vi "Open file in table.vi"() -> (0 "Error Out":errorcluster, 1 "Command Array":dbl[][](array[numeric]), 2 "Command Table":string[][](table), 3 "Details":string, 5 "Original Array":dbl[][](array[numeric]))   [LabVIEW 2011]
uses:
  <vilib>/Utility/file.llb/Read From Spreadsheet File (string).vi
panel:
  out "cancelled":bool
  out "Original Table":string[][](table)
  out "reversed array":i32[](array[numeric])
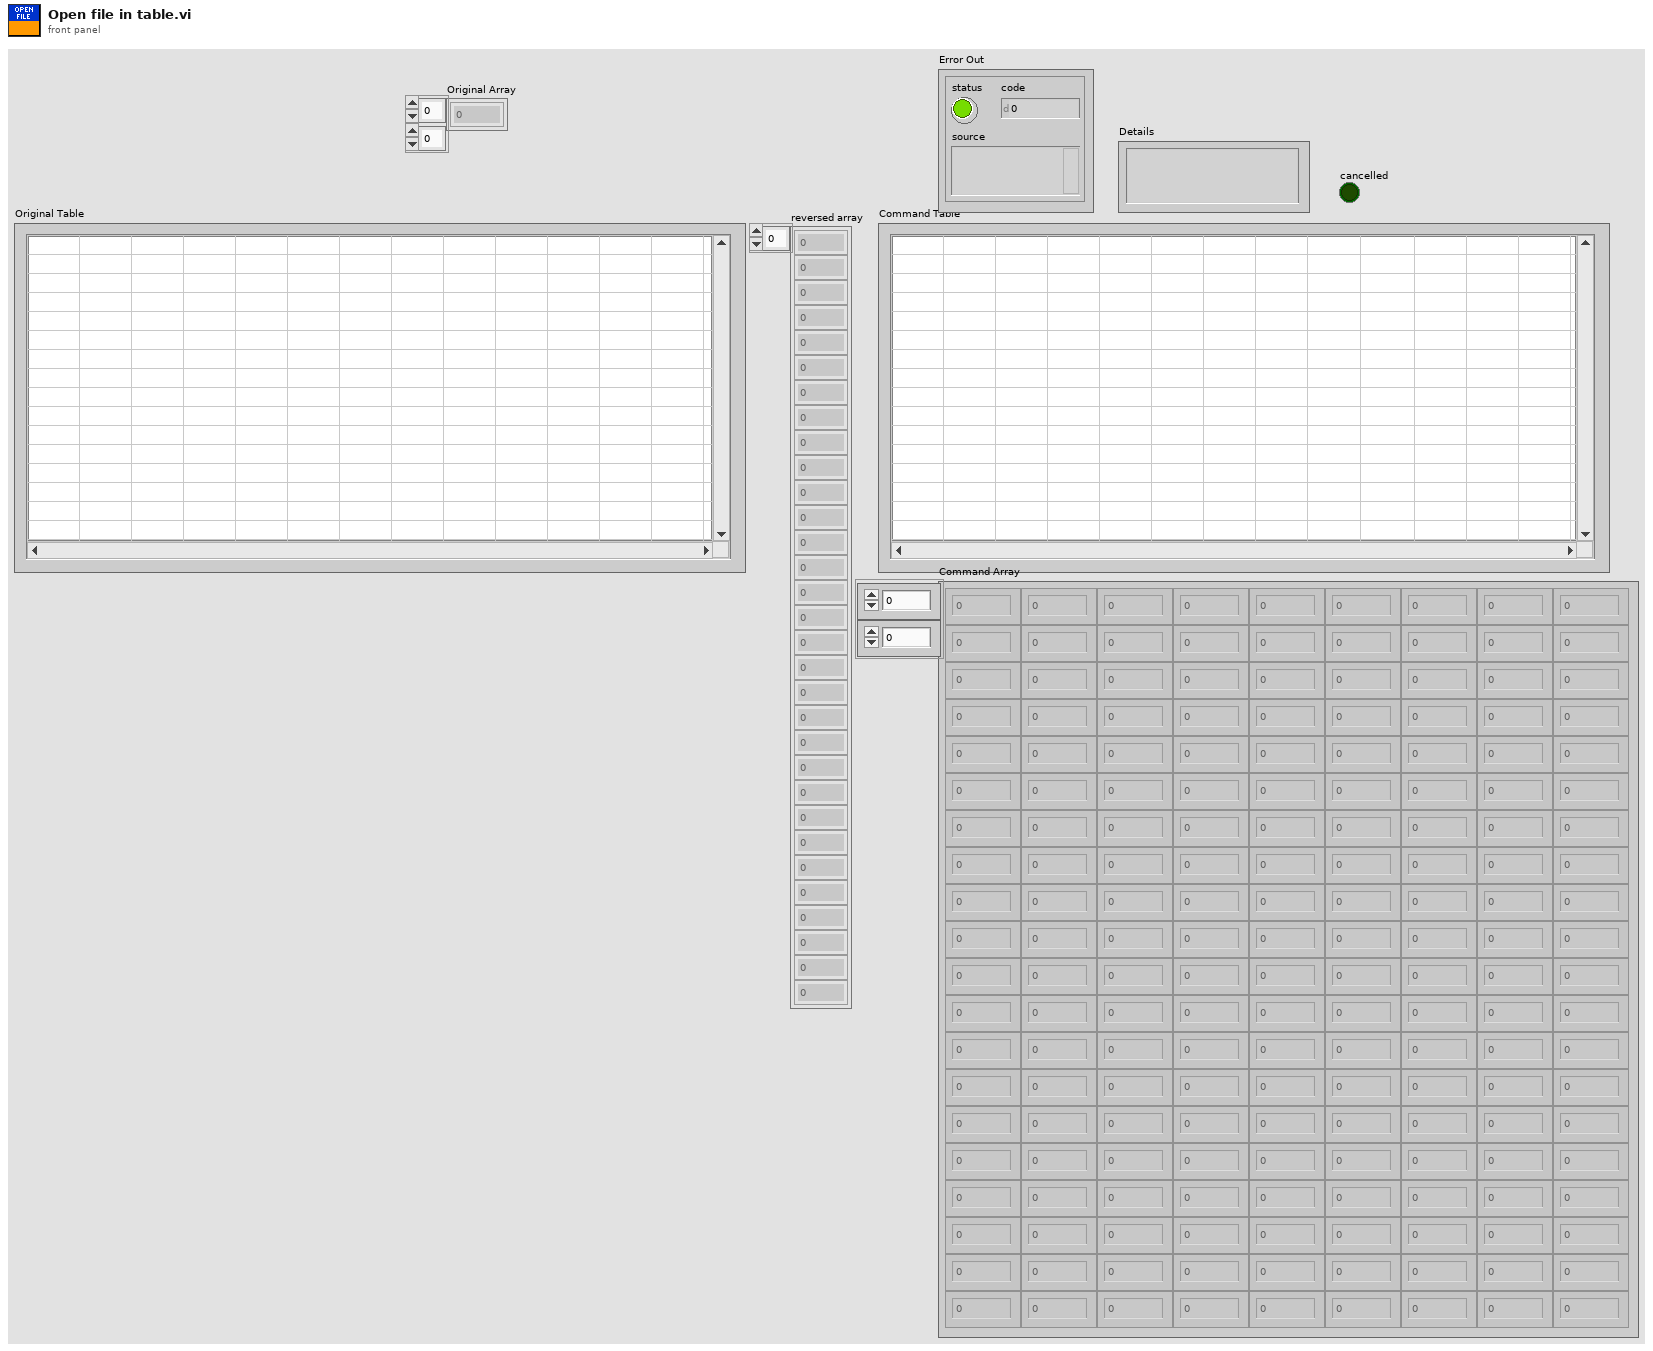
[diagram p1: front panel]
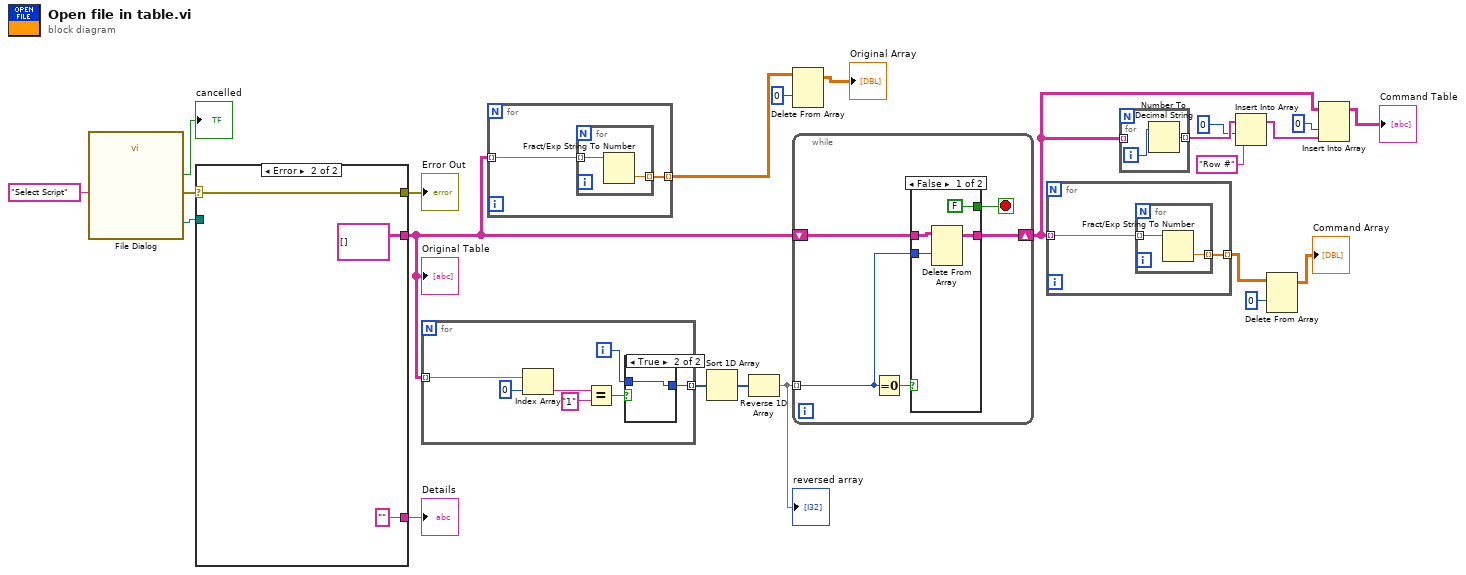
[diagram p0: block diagram]
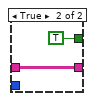
[diagram p2: hidden frame]
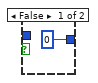
[diagram p3: hidden frame]
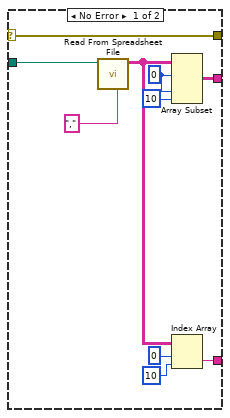
[diagram p4: hidden frame]
diagram:
  n1 = call "File Dialog"("prompt"="Select Script") -> ("selected path"=w22:path, "cancelled"=→"cancelled":bool, "error out"=w23:errorcluster)  [unwired: 11 in, 1 out]
  n2 = case shown="Error" w23 {
    selector: w23 -> [w24 w34]
    tunnel: w22 -> [w32 _]
    tunnel: [w26 string[][] []] -> w14
    tunnel: [w25 "" ("String")] -> w21
    tunnel: [w24 w34] -> w20
    frame No Error {
      w28 = 0 ("index")
      n3 = call-poly <vilib>:"Read From Spreadsheet File.vi"("delimiter (\\t)"="," ("delimiter (\\t)"), "file path (dialog if empty)"=w32) -> ("all rows"=w29:string[][])  [unwired: 5 in, 4 out]
      n4 = Array Subset(array=w29, index (row)=w28, index (col)=w28, length (col)=10 ("length")) -> (w26:string[][])  [unwired: 1 in]
      n5 = Index Array(array=w29, index (row)=0 ("disabled index (row)"), index (col)=10 ("disabled index (col)")) -> (element=w25:string)
    }
    frame Error {
    }
  }
  "Details" <- w21
  "Error Out" <- w20
  "Original Table" <- w14
  n6 = for {
    tunnel: w14 -> [w43] mode=indexing
    tunnel: [w37] -> w18 mode=indexing
    i -> [w38]
    n7 = Index Array(array=w43, index=0) -> (element=w41:string)
    n8 = Equal?(x=w41, y="1") -> (x = y?=w39:bool)
    n9 = case shown="True" w39 {
      tunnel: w38 -> [_ w45]
      tunnel: [0 w45] -> w37
      frame False {
      }
      frame True {
      }
    }
  }
  n10 = for {
    tunnel: [w47] -> w12 mode=indexing
    tunnel: w14 -> [w46] mode=indexing
    n11 = for {
      tunnel: [w49] -> w47 mode=indexing
      tunnel: w46 -> [w48] mode=indexing
      n12 = Fract/Exp String To Number(string=w48) -> (number=w49:dbl)  [unwired: 3 in, 1 out]
    }
  }
  n13 = Sort 1D Array(array=w18) -> (sorted array=w19:i32[])
  n14 = Reverse 1D Array(array=w19) -> (reversed array=w17:i32[])
  "reversed array" <- w17
  n15 = Delete From Array(array=w12, index (row)=0) -> (array with subset deleted=→"Original Array":dbl[][])  [unwired: 2 in, 1 out]
  n16 = while {
    tunnel: w17 -> [w52] mode=indexing
    shift-right: [w53] -> w7
    shift-left: w14 -> [w54]
    stop <- w50 stop-if-true
    n17 = Equal To 0?(x=w52) -> (x = 0?=w51:bool)
    n18 = case shown="False" w51 {
      tunnel: w54 -> [w58 w60]
      tunnel: [w57 w60] -> w53
      tunnel: w52 -> [w56 _]
      tunnel: [FALSE TRUE] -> w50
      frame False {
        n19 = Delete From Array(array=w58, index (row)=w56) -> (array with subset deleted=w57:string[][])  [unwired: 2 in, 1 out]
      }
      frame True {
      }
    }
  }
  n20 = for {
    tunnel: [w62] -> w9 mode=indexing
    tunnel: w7 -> [w61] mode=indexing
    n21 = for {
      tunnel: [w64] -> w62 mode=indexing
      tunnel: w61 -> [w63] mode=indexing
      n22 = Fract/Exp String To Number(string=w63) -> (number=w64:dbl)  [unwired: 3 in, 1 out]
    }
  }
  n23 = for {
    tunnel: w7 -> [_] mode=indexing
    tunnel: [w65] -> w3 mode=indexing
    i -> [w66]
    n24 = Number To Decimal String(number=w66) -> (decimal integer string=w65:string)  [unwired: 1 in]
  }
  n25 = Insert Into Array(array=w3, index=0, new element="Row #" ("new element/subarray")) -> (w4:string[])
  n26 = Delete From Array(array=w9, index (row)=0) -> (array with subset deleted=→"Command Array":dbl[][])  [unwired: 2 in, 1 out]
  n27 = Insert Into Array(array=w7, index (col)=0 ("disabled index (col)"), new element=w4) -> (→"Command Table":string[][])  [unwired: 1 in]
